vi "dfd_Convert TF Coefficients for Rendering.vi"(7 "display format":T3 items=["normal", "SOS "], 11 "filter coef":T1={"type"=enum."Undefined", "gain"=1.0, "coef a (k)"=[], "coef b (v)"=[]}) -> (0 "gain":dbl, 1 "denominator array":dbl[][](array[numeric]), 3 "numerator array":dbl[][](array[numeric]))   [LabVIEW 2017, in "NI_DigFilter_Process.lvlib"]
uses:
  <vilib>/addons/Digital Filter Design/NI_DigFilter_Process.lvlib
  <vilib>/addons/Digital Filter Design/Render.llb/dfd_Display Format.ctl
  <vilib>/addons/Digital Filter Design/_Objects.llb/DFD Filter Coef.ctl
  <vilib>/addons/Digital Filter Design/_Objects.llb/DFD Filter Structure Type Selector.ctl
  <vilib>/addons/Digital Filter Design/NI_DigFilterLicensed.lvlib
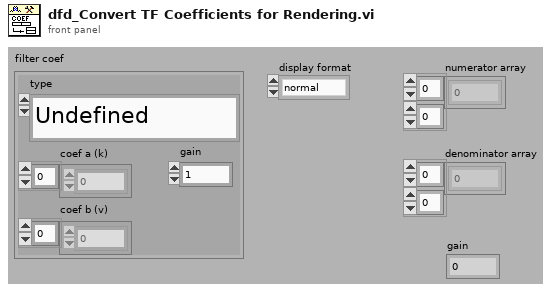
[diagram p1: front panel]
types:
  T1 = typedef "NI_DigFilterLicensed.lvlib/DFD Filter Coef.ctl" = cluster{"type":T2, "gain":dbl, "coef a (k)":dbl[], "coef b (v)":dbl[]}
  T2 = typedef "NI_DigFilterLicensed.lvlib/DFD Filter Structure Type Selector.ctl" = enum16{"Undefined", "FIR Direct Form", "FIR Direct Form Transposed", "FIR Symmetric", "FIR Antisymmetric", "IIR Direct Form I", "IIR Direct Form I Transposed", "IIR Direct Form II", "IIR Direct Form II Transposed", "IIR Cascaded Second Order Sections Form I", "IIR Cascaded Second Order Sections Form I Transposed", "IIR Cascaded Second Order Sections Form II", "IIR Cascaded Second Order Sections Form II Transposed", "Lattice Allpass (basic sections)", "Lattice Allpass (one multiplier sections)", "Lattice Allpass (normalized sections)", "Lattice AR (basic sections)", "Lattice AR (one multiplier sections)", "Lattice AR (normalized sections)", "Lattice MA (minimum phase)", "Lattice MA (maximum phase)", "Lattice ARMA (basic sections)", "Lattice ARMA (one multiplier sections)", "Lattice ARMA (normalized sections)"}
  T3 = typedef "dfd_Display Format.ctl" = u16
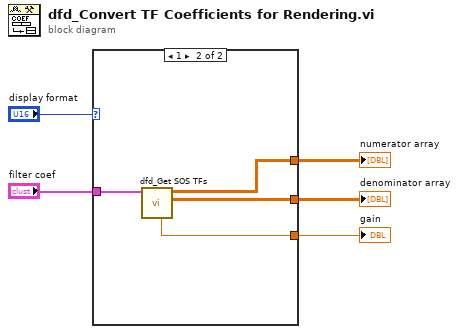
[diagram p0: block diagram]
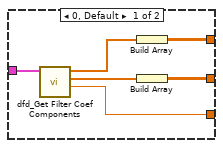
[diagram p2: hidden frame]
diagram:
  n1 = case shown="1" "display format" {
    tunnel: [w11 w14] -> w4
    tunnel: [w10 w13] -> w3
    tunnel: "filter coef" -> [w9 w15]
    tunnel: [w6 w12] -> w1
    frame 0, Default {
      n2 = call <vilib>:"dfd_Get Filter Coef Components.vi"("filter coef"=w9) -> ("gain"=w6:dbl, "coef a (k)"=w7:dbl[], "coef b (v)"=w8:dbl[])  [unwired: 1 in, 7 out]
      n3 = Build Array(w8) -> (w11:dbl[][])
      n4 = Build Array(w7) -> (w10:dbl[][])
    }
    frame 1 {
      n5 = call <vilib>:"dfd_Get SOS TFs.vi"("filter coef"=w15) -> ("dens"=w13:dbl[][], "nums"=w14:dbl[][], "gain"=w12:dbl)  [unwired: 1 in, 7 out]
    }
  }
  "numerator array" <- w4
  "denominator array" <- w3
  "gain" <- w1
